vi "Draw Compass Rose.vi"(7 "heading (rad)":dbl, 9 "draw options":T1={"Outer Border Color"=0, "Inner Border Color"=6316128, "Outer Gradient Color"=2565927, "Inner Gradient Color"=16860, "Compass North Pointer Color"=16711680, "Compass Pointer Color 1"=13355429, "Compass Pointer Color 2"=14934973, "Direction Pointer Color"=16765184, "Text Box Outline Color"=13355429, "Text Box Background Color"=14934973, "Scale Color"=16448250, "Text Color"=0, "Draw Gradient"=TRUE, "Draw Rose"=TRUE, "Simple Scale"=TRUE, "Draw Text"=FALSE, "Font Name"="Helvetica", "Angle Units"=enum."Degrees"}, 10 "draw area cache in":T3, 11 "picture in":picture) -> (3 "picture out":picture)   [LabVIEW 2017, in "NI_Robotics_Compass Picture.lvlib"]
uses:
  <vilib>/robotics/Controls/Compass Indicator/Compass Picture/NI_Robotics_Compass Picture.lvlib
  <vilib>/robotics/Controls/Compass Indicator/Compass Picture/Draw Area State.ctl
  <vilib>/Utility/miscctls.llb/LVBoundsTypeDef.ctl
  <vilib>/robotics/Controls/Compass Indicator/Compass Picture/Draw Options.ctl
  <vilib>/robotics/Controls/Utilities/Angle Units.ctl
  <vilib>/picture/picture.llb/Draw Multiple Lines.vi
  <vilib>/picture/pictutil.llb/Hilite Color.vi
  <vilib>/Utility/AngleManip/Degrees to Radians (Array DBL).vi
  <vilib>/Utility/AngleManip/Degrees to Radians (Scalar DBL).vi
  <vilib>/Utility/AngleManip/NI_AngleManipulation.lvlib
  <vilib>/robotics/Controls/Utilities/NI_Robotics_Control Utilities.lvlib
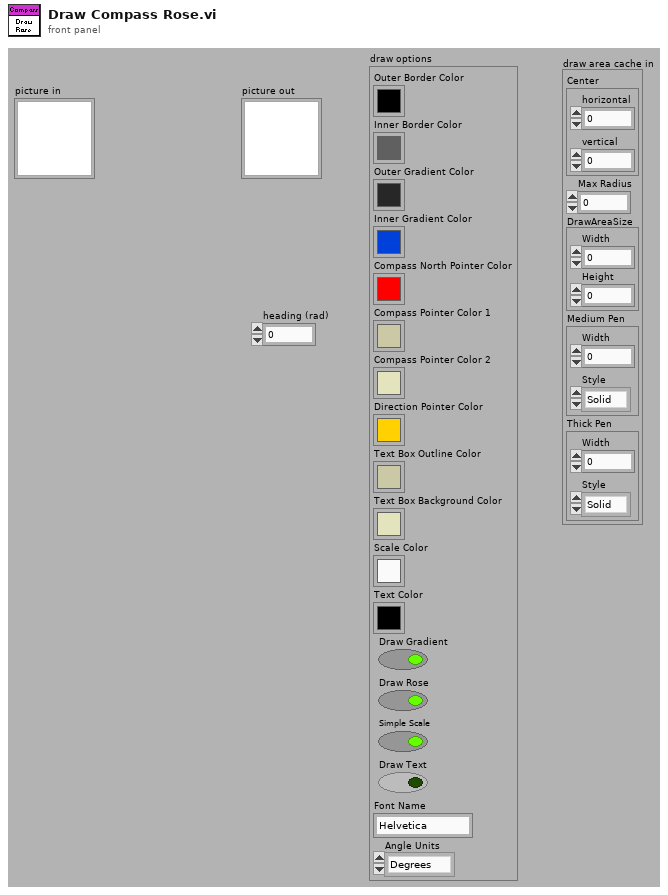
[diagram p1: front panel]
types:
  T1 = typedef "NI_Robotics_Compass Picture.lvlib/Draw Options.ctl" = cluster{"Outer Border Color":u32, "Inner Border Color":u32, "Outer Gradient Color":u32, "Inner Gradient Color":u32, "Compass North Pointer Color":u32, "Compass Pointer Color 1":u32, "Compass Pointer Color 2":u32, "Direction Pointer Color":u32, "Text Box Outline Color":u32, "Text Box Background Color":u32, "Scale Color":u32, "Text Color":u32, "Draw Gradient":bool, "Draw Rose":bool, "Simple Scale":bool, "Draw Text":bool, "Font Name":string, "Angle Units":T2}
  T2 = typedef "NI_Robotics_Control Utilities.lvlib/Angle Units.ctl" = enum16{"Radians", "Degrees"}
  T3 = typedef "NI_Robotics_Compass Picture.lvlib/Draw Area State.ctl" = cluster{"Center":cluster{"horizontal":i16, "vertical":i16}, "Max Radius":dbl, "DrawAreaSize":T4, "Medium Pen":cluster{"Width":u16, "Style":enum32{"Solid", "Dash", "Dot", "DashDot", "DashDotDot"}}, "Thick Pen":cluster{"Width":u16, "Style":enum32{"Solid", "Dash", "Dot", "DashDot", "DashDotDot"}}}
  T4 = typedef "LVBoundsTypeDef.ctl" = cluster{"Width":u32, "Height":u32}
  T5 = cluster{"Width":u16, "Style":enum32{"Solid", "Dash", "Dot", "DashDot", "DashDotDot"}}
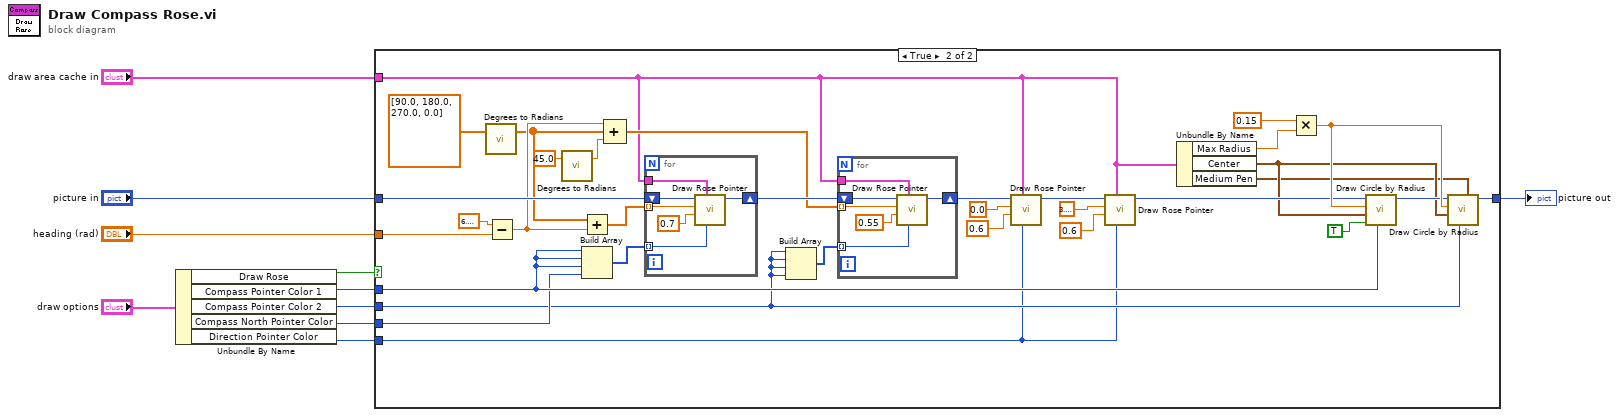
[diagram p0: block diagram]
diagram:
  n1 = Unbundle By Name("draw options") -> ("Draw Rose"=w5:bool, "Compass Pointer Color 1"=w4:u32, "Compass Pointer Color 2"=w3:u32, "Compass North Pointer Color"=w2:u32, "Direction Pointer Color"=w1:u32)
  n2 = case shown="True" w5 {
    tunnel: [w11 w41] -> w10
    tunnel: "picture in" -> [w11 w36]
    tunnel: "heading (rad)" -> [_ w26]
    tunnel: "draw area cache in" -> [_ w23]
    tunnel: w4 -> [_ w15]
    tunnel: w3 -> [_ w13]
    tunnel: w2 -> [_ w14]
    tunnel: w1 -> [_ w12]
    frame False {
    }
    frame True {
      n3 = call-poly <vilib>:"Degrees to Radians.vi"("angles (deg)"=dbl[] [90.0, 180.0, 270.0, 0.0]) -> ("angles (rad)"=w18:dbl[])  [unwired: 2 in]
      n4 = Subtract(x=6.283185307179586, y=w26) -> (x-y=w25:dbl)
      n5 = call-poly <vilib>:"Degrees to Radians.vi"("angle (deg)"=45.0 ("Rose Size (0-1)")) -> ("angle (rad)"=w16:dbl)  [unwired: 2 in]
      n6 = Add(x=w18, y=w25) -> (x+y=w34:dbl[])
      n7 = Build Array(w15, w15, w15, w14) -> (w43:u32[])
      n8 = Compound Arithmetic op=ADD(w25, w18, w16) -> (w35:dbl[])
      n9 = for {
        shift-right: [w55] -> w37
        shift-left: w36 -> [w56]
        tunnel: w43 -> [w54] mode=indexing
        tunnel: w34 -> [w53] mode=indexing
        tunnel: w23 -> [w51]
        n10 = call <vilib>:"Draw Rose Pointer.vi"("compass pointer color"=w54, "draw area cache"=w51, "rose size (0-1)"=0.7 ("Rose Size (0-1)"), "heading (rad)"=w53, "picture in"=w56) -> ("picture out"=w55:picture)  [unwired: 6 in]
      }
      n11 = Build Array(w13, w13, w13, w13) -> (w44:u32[])
      n12 = for {
        shift-right: [w49] -> w33
        shift-left: w37 -> [w50]
        tunnel: w44 -> [w48] mode=indexing
        tunnel: w35 -> [w47] mode=indexing
        tunnel: w23 -> [w45]
        n13 = call <vilib>:"Draw Rose Pointer.vi"("compass pointer color"=w48, "draw area cache"=w45, "rose size (0-1)"=0.55 ("Rose Size (0-1)"), "heading (rad)"=w47, "picture in"=w50) -> ("picture out"=w49:picture)  [unwired: 6 in]
      }
      n14 = call <vilib>:"Draw Rose Pointer.vi"("compass pointer color"=w12, "draw area cache"=w23, "rose size (0-1)"=0.6 ("Rose Size (0-1)"), "heading (rad)"=0.0 ("Heading (degrees)"), "picture in"=w33) -> ("picture out"=w30:picture)  [unwired: 6 in]
      n15 = call <vilib>:"Draw Rose Pointer.vi"("compass pointer color"=w12, "draw area cache"=w23, "rose size (0-1)"=0.6 ("Rose Size (0-1)"), "heading (rad)"=3.141592653589793 ("Heading (degrees)"), "picture in"=w30) -> ("picture out"=w29:picture)  [unwired: 6 in]
      n16 = Unbundle By Name(w23) -> ("Max Radius"=w21:dbl, "Center"=w22:cluster{"horizontal":i16, "vertical":i16}, "Medium Pen"=w20:T5)
      n17 = Multiply(x=0.15 ("Rose Size (0-1)"), y=w21) -> (x*y=w42:dbl)
      n18 = call <vilib>:"Draw Circle by Radius.vi"("color(black)"=w15, "fill?(F)"=TRUE, "pixel center"=w22, "radius"=w42, "picture"=w29) -> ("new picture"=w40:picture)  [unwired: 6 in]
      n19 = call <vilib>:"Draw Circle by Radius.vi"("pen"=w20, "color(black)"=w13, "pixel center"=w22, "radius"=w42, "picture"=w40) -> ("new picture"=w41:picture)  [unwired: 6 in]
    }
  }
  "picture out" <- w10
